vi "Compute New Configuration File MD5 and Compare.vi"(8 "error in (no error)":errorcluster, 10 "New Path File":path, 11 "CD Ref In":T1=18446744073709551615 format="%.0x") -> (0 "error out":errorcluster, 2 "MD5 message-digest":string, 3 "MD5 Changed?":bool)   [LabVIEW 2013, in "Modbus System Explorer.lvlib"]
uses:
  Modbus System Explorer.lvlib
  <vilib>/NI Veristand/Custom Device API/Custom Device Item Ref.ctl
  Glyphs/Modbus Property Names.vi
  <vilib>/NI Veristand/Custom Device API/Get Item Property (String).vi
  Shared/Modbus Shared.lvlib
  <vilib>/NI Veristand/Custom Device API/Custom Device API.lvlib
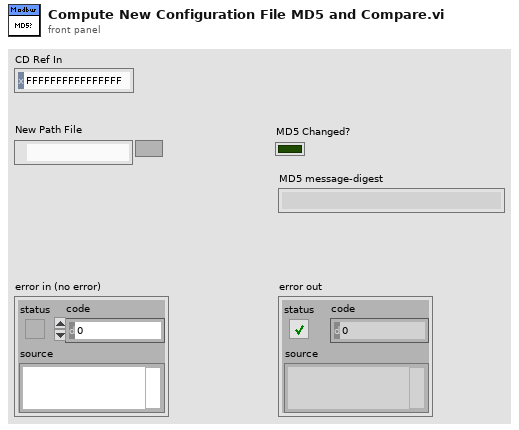
[diagram p1: front panel]
types:
  T1 = typedef "Custom Device API.lvlib/Custom Device Item Ref.ctl" = u64
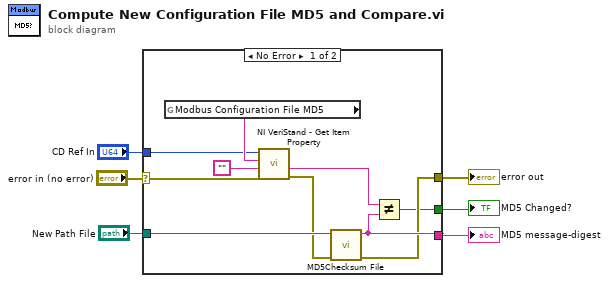
[diagram p0: block diagram]
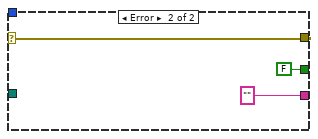
[diagram p2: hidden frame]
diagram:
  n1 = case shown="No Error" "error in (no error)" {
    selector: "error in (no error)" -> [w12 w19]
    tunnel: "New Path File" -> [w16 _]
    tunnel: "CD Ref In" -> [w13 _]
    tunnel: [w8 w19] -> w3
    tunnel: [w9 "" ("MD5 message-digest")] -> w2
    tunnel: [w7 FALSE] -> w1
    frame No Error {
      n2 = global read "Modbus Property Names.vi" "Modbus Configuration File MD5"() -> (w15:string)
      n3 = call-poly <vilib>:"NI VeriStand - Get Item Property.vi"("error in (no error)"=w12, "Default Value"="", "Property Name"=w15, "Item Ref in"=w13) -> ("error out"=w11:errorcluster, "Value"=w10:string)  [unwired: 4 in, 2 out]
      n4 = call <vilib>:"MD5Checksum File.vi"("error in (no error)"=w11, "Path"=w16) -> ("error out"=w8:errorcluster, "MD5 message-digest"=w9:string)  [unwired: 8 in]
      n5 = Not Equal?(x=w10, y=w9) -> (x != y?=w7:bool)
    }
    frame Error {
    }
  }
  "MD5 Changed?" <- w1
  "MD5 message-digest" <- w2
  "error out" <- w3
